vi "CTUD.vi"(0 "CTU":bool, 1 "CTD":bool, 2 "PV":i32, 3 "Reset":bool) -> (14 "Q":bool, 15 "CT":i32)   [LabVIEW 2020]
uses:
  7b58aaaf-3230-4726-a54c-2c8544926117.vi
panel:
  out "Mem2":bool
  out "Mem":bool
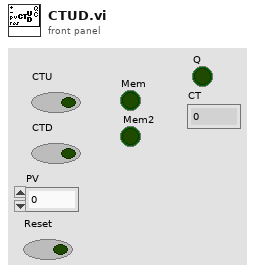
[diagram p1: front panel]
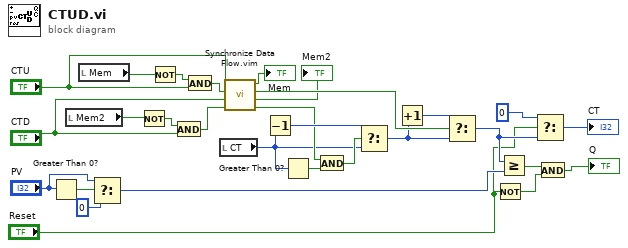
[diagram p0: block diagram]
diagram:
  n1 = Greater Than 0?(x="PV") -> (x > 0?=w29:bool)
  n2 = local read "Mem2"() -> (w8:bool)
  n3 = local read "Mem"() -> (w19:bool)
  n4 = Select(t="PV", s=w29, f=0) -> (s? t:f=w21:i32)
  n5 = Not(x=w8) -> (.not. x?=w11:bool)
  n6 = Not(x=w19) -> (.not. x?=w20:bool)
  n7 = And(x=w11, y="CTD") -> (x .and. y?=w7:bool)
  n8 = And(x=w20, y="CTU") -> (x .and. y?=w26:bool)
  n9 = local read "CT"() -> (w1:i32)
  n10 = call "Synchronize Data Flow.vim"("input 4"=w7, "input 3"="CTD", "input 2"=w26, "input 1"="CTU") -> ("output 4"=w2:bool, "output 3"=→"Mem2":bool, "output 2"=w23:bool, "output 1"=→"Mem":bool)
  n11 = Decrement(x=w1) -> (x-1=w6:i32)
  n12 = Greater Than 0?(x=w1) -> (x > 0?=w4:bool)
  n13 = And(x=w2, y=w4) -> (x .and. y?=w3:bool)
  n14 = Select(t=w6, s=w3, f=w1) -> (s? t:f=w5:i32)
  n15 = Increment(x=w5) -> (x+1=w22:i32)
  n16 = Select(t=w22, s=w23, f=w5) -> (s? t:f=w15:i32)
  n17 = Not(x="Reset") -> (.not. x?=w16:bool)
  n18 = Greater Or Equal?(x=w15, y=w21) -> (x >= y?=w18:bool)
  n19 = Select(t=0, s="Reset", f=w15) -> (s? t:f=→"CT":i32)
  n20 = And(x=w18, y=w16) -> (x .and. y?=→"Q":bool)
